vi "Zad3_kolokwium_nie_oddane_fuck.vi"() -> ()   [LabVIEW 2020]
panel:
  in  "stop":bool
  out "Losowana liczba co sekundê":string
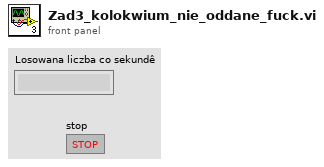
[diagram p1: front panel]
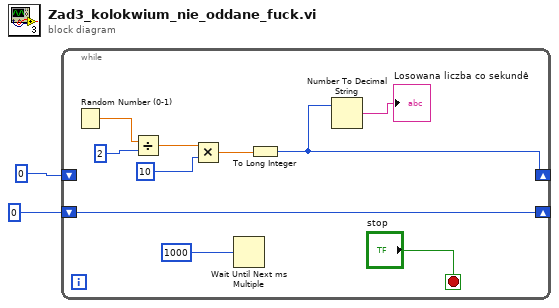
[diagram p0: block diagram]
diagram:
  n1 = while {
    shift-right: [w7] -> _
    shift-left: 0 -> [_]
    shift-right: [w3] -> _
    shift-left: 0 -> [w3]
    stop <- "stop" stop-if-true
    n2 = Random Number (0-1)() -> (number: 0 to 1=w12:dbl)
    n3 = Divide(x=w12, y=2) -> (x/y=w11:dbl)
    n4 = Multiply(x=w11, y=10) -> (x*y=w10:dbl)
    n5 = Wait Until Next ms Multiple(millisecond multiple=1000) -> ()  [unwired: 1 out]
    n6 = To Long Integer(number=w10) -> (32bit integer=w7:i32)
    n7 = Number To Decimal String(number=w7) -> (decimal integer string=→"Losowana liczba co sekundê":string)  [unwired: 1 in]
  }
